vi "Read with parameters.vi"(8 "error in (no error)":errorcluster, 11 "pcap reference in":u32) -> (0 "error out":errorcluster, 2 "capture_data out":string, 3 "pcap reference out":u32)   [LabVIEW 2017]
uses:
  Lib/WinPcap/lvwpcap.lvlib
panel:
  out "timed out":bool
  out "timestamp":cluster{"tv_sec":u32, "tv_usec":u32}
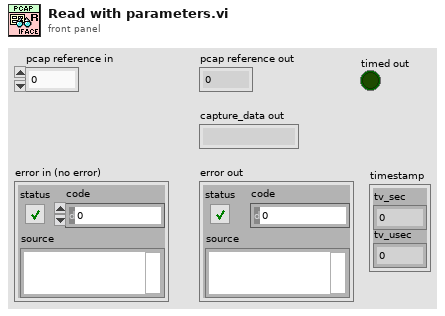
[diagram p1: front panel]
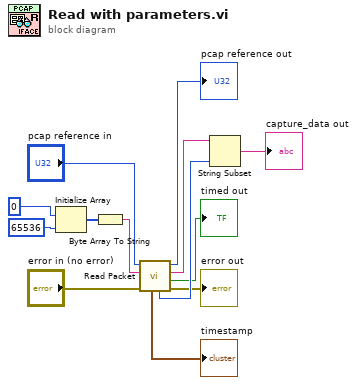
[diagram p0: block diagram]
diagram:
  n1 = Initialize Array(u8 0, 65536 ("capture_size (65536)")) -> (w9:u8[])
  n2 = Byte Array To String(unsigned byte array=w9) -> (string=w11:string)
  n3 = call "Read Packet.vi"("error in (no error)"="error in (no error)", "capture_data"=w11, "pcap reference"="pcap reference in") -> ("error out"=→"error out":errorcluster, "timed out"=→"timed out":bool, "capture_data out"=w7:string, "pcap reference out"=→"pcap reference out":u32, "capture_len"=w8:u32, "timestamp"=→"timestamp":cluster{"tv_sec":u32, "tv_usec":u32})  [unwired: 3 in]
  n4 = String Subset(string=w7, length (rest)=w8) -> (substring=→"capture_data out":string)  [unwired: 1 in]
